vi "MessageName.vi"(11 "Message in":refnum<class "Message.lvclass">) -> (2 "MessageName":string)   [LabVIEW 2020, in "LV-Proto.lvlib" / "Message.lvclass"]
uses:
  Message.lvclass
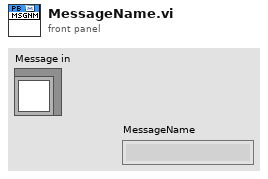
[diagram p1: front panel]
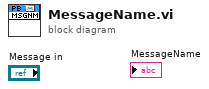
[diagram p0: block diagram]
diagram:
